vi "Sample-Encoder conversion.vi"(6 "Encoder Position":i32, 7 "Step Window radius":i32, 10 "New Sample Number":i16, 11 "Encoder offset":i16) -> (1 "Encoder destination":i32, 2 "Within Range?":bool, 3 "Encoder displacement":i32)   [LabVIEW 2016]
doc: "Sample-Encoder conversion\n\nInputs\nEncoder offset - encoder position of wheel zero (sample #1)\nNew Sample Number - requested sample number\nEncoder Position - current position of wheel in encoder units\nStep Window radius - how precise should the move be\n\nOutputs\nEncoder Destination - Requested sample number mapped to encoder position\nWithin Rnage? - Boolean\nEncoder Displacement - how far to move and in what direction\n\nMethod\n1. Map New Sample Number to encoder position accounting for offset and \"rollover\" \n\n2. Calculate shortest distance between target position and current position - 2 cases: 1 direct route and 2 crossing the rollover point. NOTE: There are issues with signs and directions of rotation that were worked out by trail and error\n\n3. Compare to limit - how precise do we need the wheel's position to be -- is it within range?\n\n4. Output displacement of the shortest move and within range"
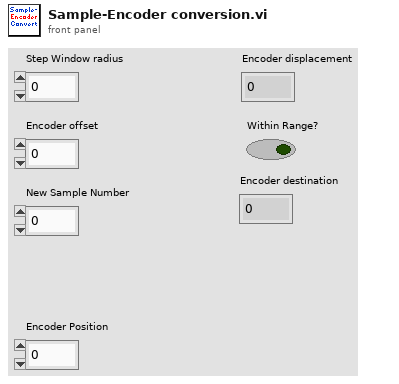
[diagram p1: front panel]
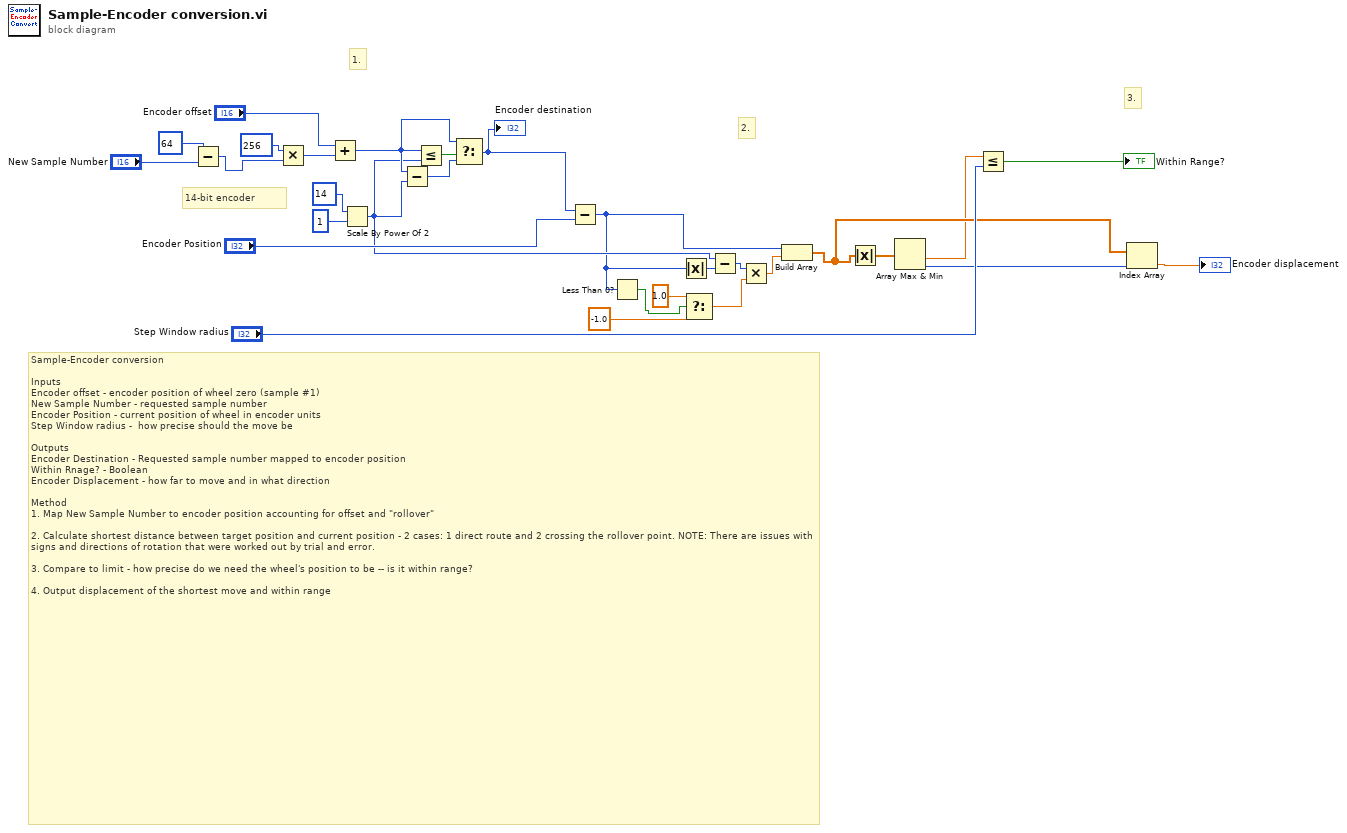
[diagram p0: block diagram]
diagram:
  # "3."
  # "2."
  # "1."
  # "Sample-Encoder conversion\n\nInputs\nEncoder offset - encoder position of wheel zero (sample #1)\nNew Sample Number - requested sample number\nEncoder Position - current position of wheel in encoder units\nStep Window radius -  how precise should the move be\n\nOutputs\nEncoder Destination - Requested sample number mapped to encoder position\nWithin Rnage? - Boolean\nEncoder Displacement - how far to move and in what direction\n\nMethod\n1. Map New Sample Number to encoder position accounting for offset and \"rollover\" \n\n2. Calculate shortest distance between target position and current position - 2 cases: 1 direct route and 2 crossing the rollover point. NOTE: There are issues with signs and directions of rotation that were worked out by trial and error.\n\n3. Compare to limit - how precise do we need the wheel's position to be -- is it within range?\n\n4. Output displacement of the shortest move and within range"
  # "14-bit encoder"
  n1 = Subtract(x=i16 64, y="New Sample Number") -> (x-y=w10:i16)
  n2 = Multiply(x=i16 256, y=w10) -> (x*y=w28:i16)
  n3 = Add(x="Encoder offset", y=w28) -> (x+y=w19:i16)
  n4 = Scale By Power Of 2(n=i16 14, x=i16 1) -> (x*2^n=w16:i16)
  n5 = Subtract(x=w19, y=w16) -> (x-y=w20:i16)
  n6 = Less Or Equal?(x=w19, y=w16) -> (x <= y?=w21:bool)
  n7 = Select(t=w19, s=w21, f=w20) -> (s? t:f=w18:i16)
  "Encoder destination" <- w18
  n8 = Subtract(x=w18, y="Encoder Position") -> (x-y=w1:i32)
  n9 = Less Than 0?(x=w1) -> (x < 0?=w2:bool)
  n10 = Absolute Value(x=w1) -> (abs(x)=w8:i32)
  n11 = Select(t=1.0, s=w2, f=-1.0) -> (s? t:f=w5:dbl)
  n12 = Subtract(x=w16, y=w8) -> (x-y=w6:i32)
  n13 = Multiply(x=w6, y=w5) -> (x*y=w7:dbl)
  n14 = Build Array(w1, w7) -> (w13:dbl[])
  n15 = Absolute Value(x=w13) -> (abs(x)=w15:dbl[])
  n16 = Array Max & Min(array=w15) -> (min value=w11:dbl, min index (indices)=w14:i32)  [unwired: 2 out]
  n17 = Less Or Equal?(x=w11, y="Step Window radius") -> (x <= y?=→"Within Range?":bool)
  n18 = Index Array(array=w13, index=w14) -> (element=→"Encoder displacement":dbl)
